vi "Turn On.vi"(0 "Interface_object in":refnum<class "Lamp.lvclass">, 5 "error in (no error)":errorcluster) -> (14 "Interface_object out":refnum<class "Lamp.lvclass">, 19 "error out":errorcluster)   [LabVIEW 2018, in "Lamp.lvclass"]
uses:
  Lamp.lvclass
  Lamp.lvclass/Lamp.ctl
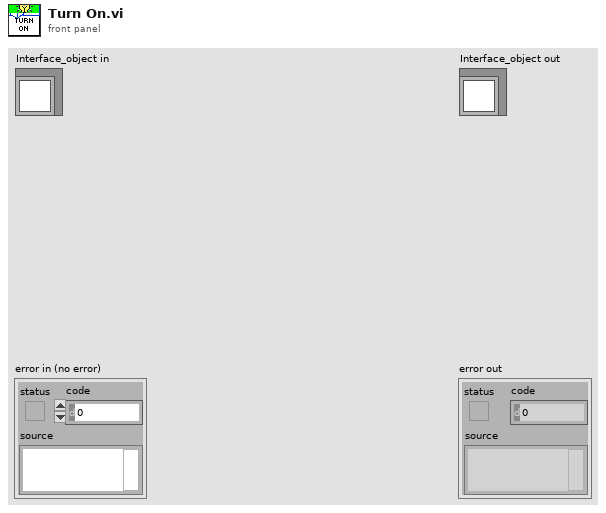
[diagram p1: front panel]
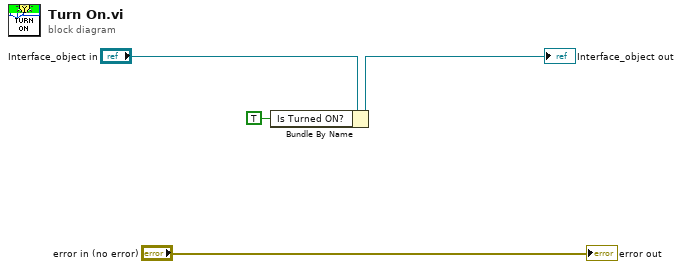
[diagram p0: block diagram]
diagram:
  n1 = Bundle By Name(cluster="Interface_object in", "Is Turned ON?"=TRUE) -> (→"Interface_object out":refnum<class "Lamp.lvclass">)
  "error out" <- "error in (no error)"
